vi "write_command.vi"(8 "error in (no error)":errorcluster, 9 "read (T)":bool=TRUE, 10 "string to write":string, 11 "LightSourceAN191011Chameleon in":refnum<class "LightSourceAN191011Chameleon.lvclass">) -> (0 "error out":errorcluster, 2 "read string":string, 3 "LightSourceAN191011Chameleon out":refnum<class "LightSourceAN191011Chameleon.lvclass">)   [LabVIEW 2010, in "LightSourceAN191011Chameleon.lvclass"]
uses:
  LightSourceAN191011Chameleon.lvclass
  LightSourceAN191011Chameleon.lvclass/LightSourceAN191011Chameleon.ctl
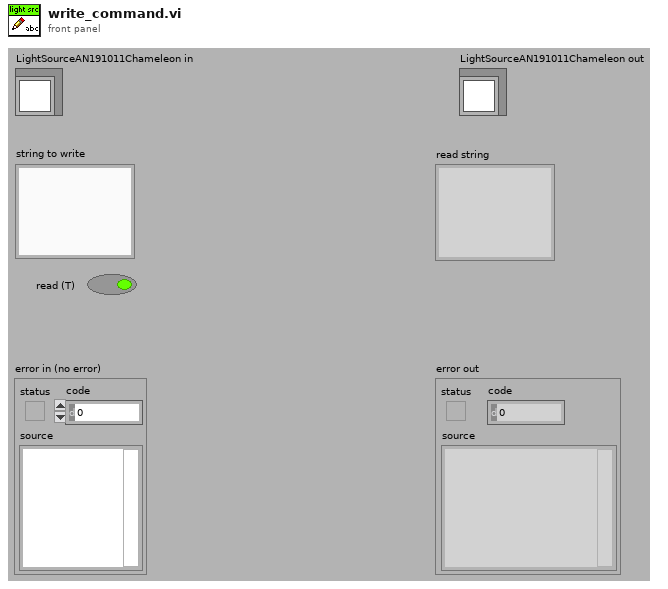
[diagram p1: front panel]
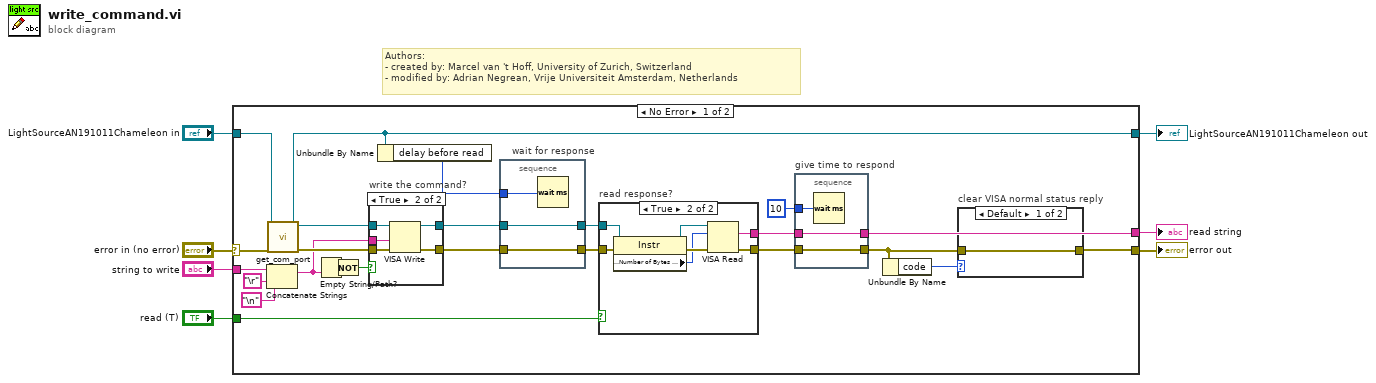
[diagram p0: block diagram]
diagram:
  # "Authors: \n- created by: Marcel van 't Hoff, University of Zurich, Switzerland\n- modified by: Adrian Negrean, Vrije Universiteit Amsterdam, Netherlands"
  n1 = case shown="No Error" "error in (no error)" {
    selector: "error in (no error)" -> [w23 w55]
    tunnel: [w10 w55] -> w6
    tunnel: [w20 w54] -> w4
    tunnel: "LightSourceAN191011Chameleon in" -> [w27 w54]
    tunnel: "string to write" -> [w31 _]
    tunnel: [w14 _] -> w2
    tunnel: "read (T)" -> [w13 _]
    frame No Error {
      n2 = Concatenate Strings(w31, "\r", "\n") -> (w24:string)
      n3 = call-dynamic "get_com_port.vi"("error in (no error)"=w23, "LightSourceAN191011Chameleon in"=w27) -> ("error out"=w26:errorcluster, "comm port"=w25:refnum<visa-resource-name>, "LightSourceAN191011Chameleon out"=w20:refnum<class "LightSourceAN191011Chameleon.lvclass">)  [unwired: 7 in]
      n4 = Empty String/Path?(string/path=w24) -> (empty?=w28:bool)
      n5 = Not(x=w28) -> (.not. x?=w12:bool)
      n6 = case "write the command?" shown="True" w12 {
        tunnel: [w47 w53] -> w21
        tunnel: [w48 w52] -> w22
        tunnel: w26 -> [w47 w51]
        tunnel: w25 -> [w48 w50]
        tunnel: w24 -> [_ w49]
        frame False {
        }
        frame True {
          n7 = VISA Write(VISA resource name=w50, write buffer=w49, error in (no error)=w51) -> (VISA resource name out=w52:refnum<visa-resource-name>, error out=w53:errorcluster)  [unwired: 1 out]
        }
      }
      n8 = Unbundle By Name(w20) -> ("delay before read"=w8:u32)
      n9 = stacked-sequence "wait for response" {
        tunnel: w21 -> [w46]
        tunnel: [w46] -> w15
        tunnel: w22 -> [w45]
        tunnel: [w45] -> w16
        tunnel: w8 -> [w44]
        frame #0 {
          n10 = Wait (ms)(milliseconds to wait=w44) -> ()  [unwired: 1 out]
        }
      }
      n11 = case "read response?" shown="True" w13 {
        tunnel: w15 -> [w36 w40]
        tunnel: [w36 w43] -> w19
        tunnel: w16 -> [_ w42]
        tunnel: [_ w37] -> w18
        frame False {
        }
        frame True {
          n12 = property class="Instr"(reference=w42, error in=w40) -> (reference out=w41:refnum<visa-resource-name>, error out=w39:errorcluster, "Serial Settings:Number of Bytes at Serial Port"=w38:u32)
          n13 = VISA Read(VISA resource name=w41, byte count=w38, error in (no error)=w39) -> (read buffer=w37:string, error out=w43:errorcluster)  [unwired: 2 out]
        }
      }
      n14 = stacked-sequence "give time to respond" {
        tunnel: w19 -> [w35]
        tunnel: [w35] -> w11
        tunnel: w18 -> [w34]
        tunnel: [w34] -> w14
        tunnel: u32 10 ("delay before read (ms)") -> [w33]
        frame #0 {
          n15 = Wait (ms)(milliseconds to wait=w33) -> ()  [unwired: 1 out]
        }
      }
      n16 = Unbundle By Name(w11) -> ("code"=w9:i32)
      n17 = case "clear VISA normal status reply" shown="Default" w9 {
        tunnel: w11 -> [w32 _]
        tunnel: [w32 _] -> w10
        frame Default {
        }
        frame 1073676294 {
        }
      }
    }
    frame Error {
    }
  }
  "error out" <- w6
  "LightSourceAN191011Chameleon out" <- w4
  "read string" <- w2
